vi "FEA_Model_LEMP.vi"(8 "error in (no error)":errorcluster, 11 "FEA_Model in":refnum<class "FEA_Model.lvclass">) -> (0 "error out":errorcluster, 3 "FEA_Model out":refnum<class "FEA_Model.lvclass">)   [LabVIEW 2021, in "FEA_Model.lvclass"]
uses:
  FEA_Model.lvclass
  FEA_Model.lvclass/FEA_Model.ctl
panel:
  in  "Mode count":i32=3
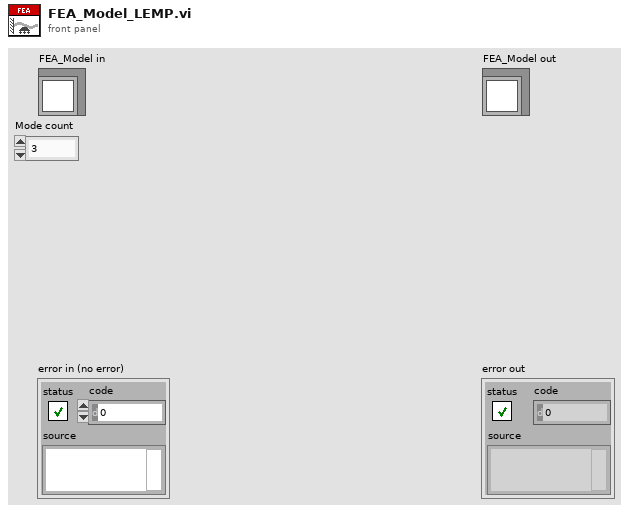
[diagram p1: front panel]
types:
  T1 = cluster{"Eigenvalues":dbl[], "SquareT Eigenvectors":dbl[][], "1/deltaStiff":dbl}
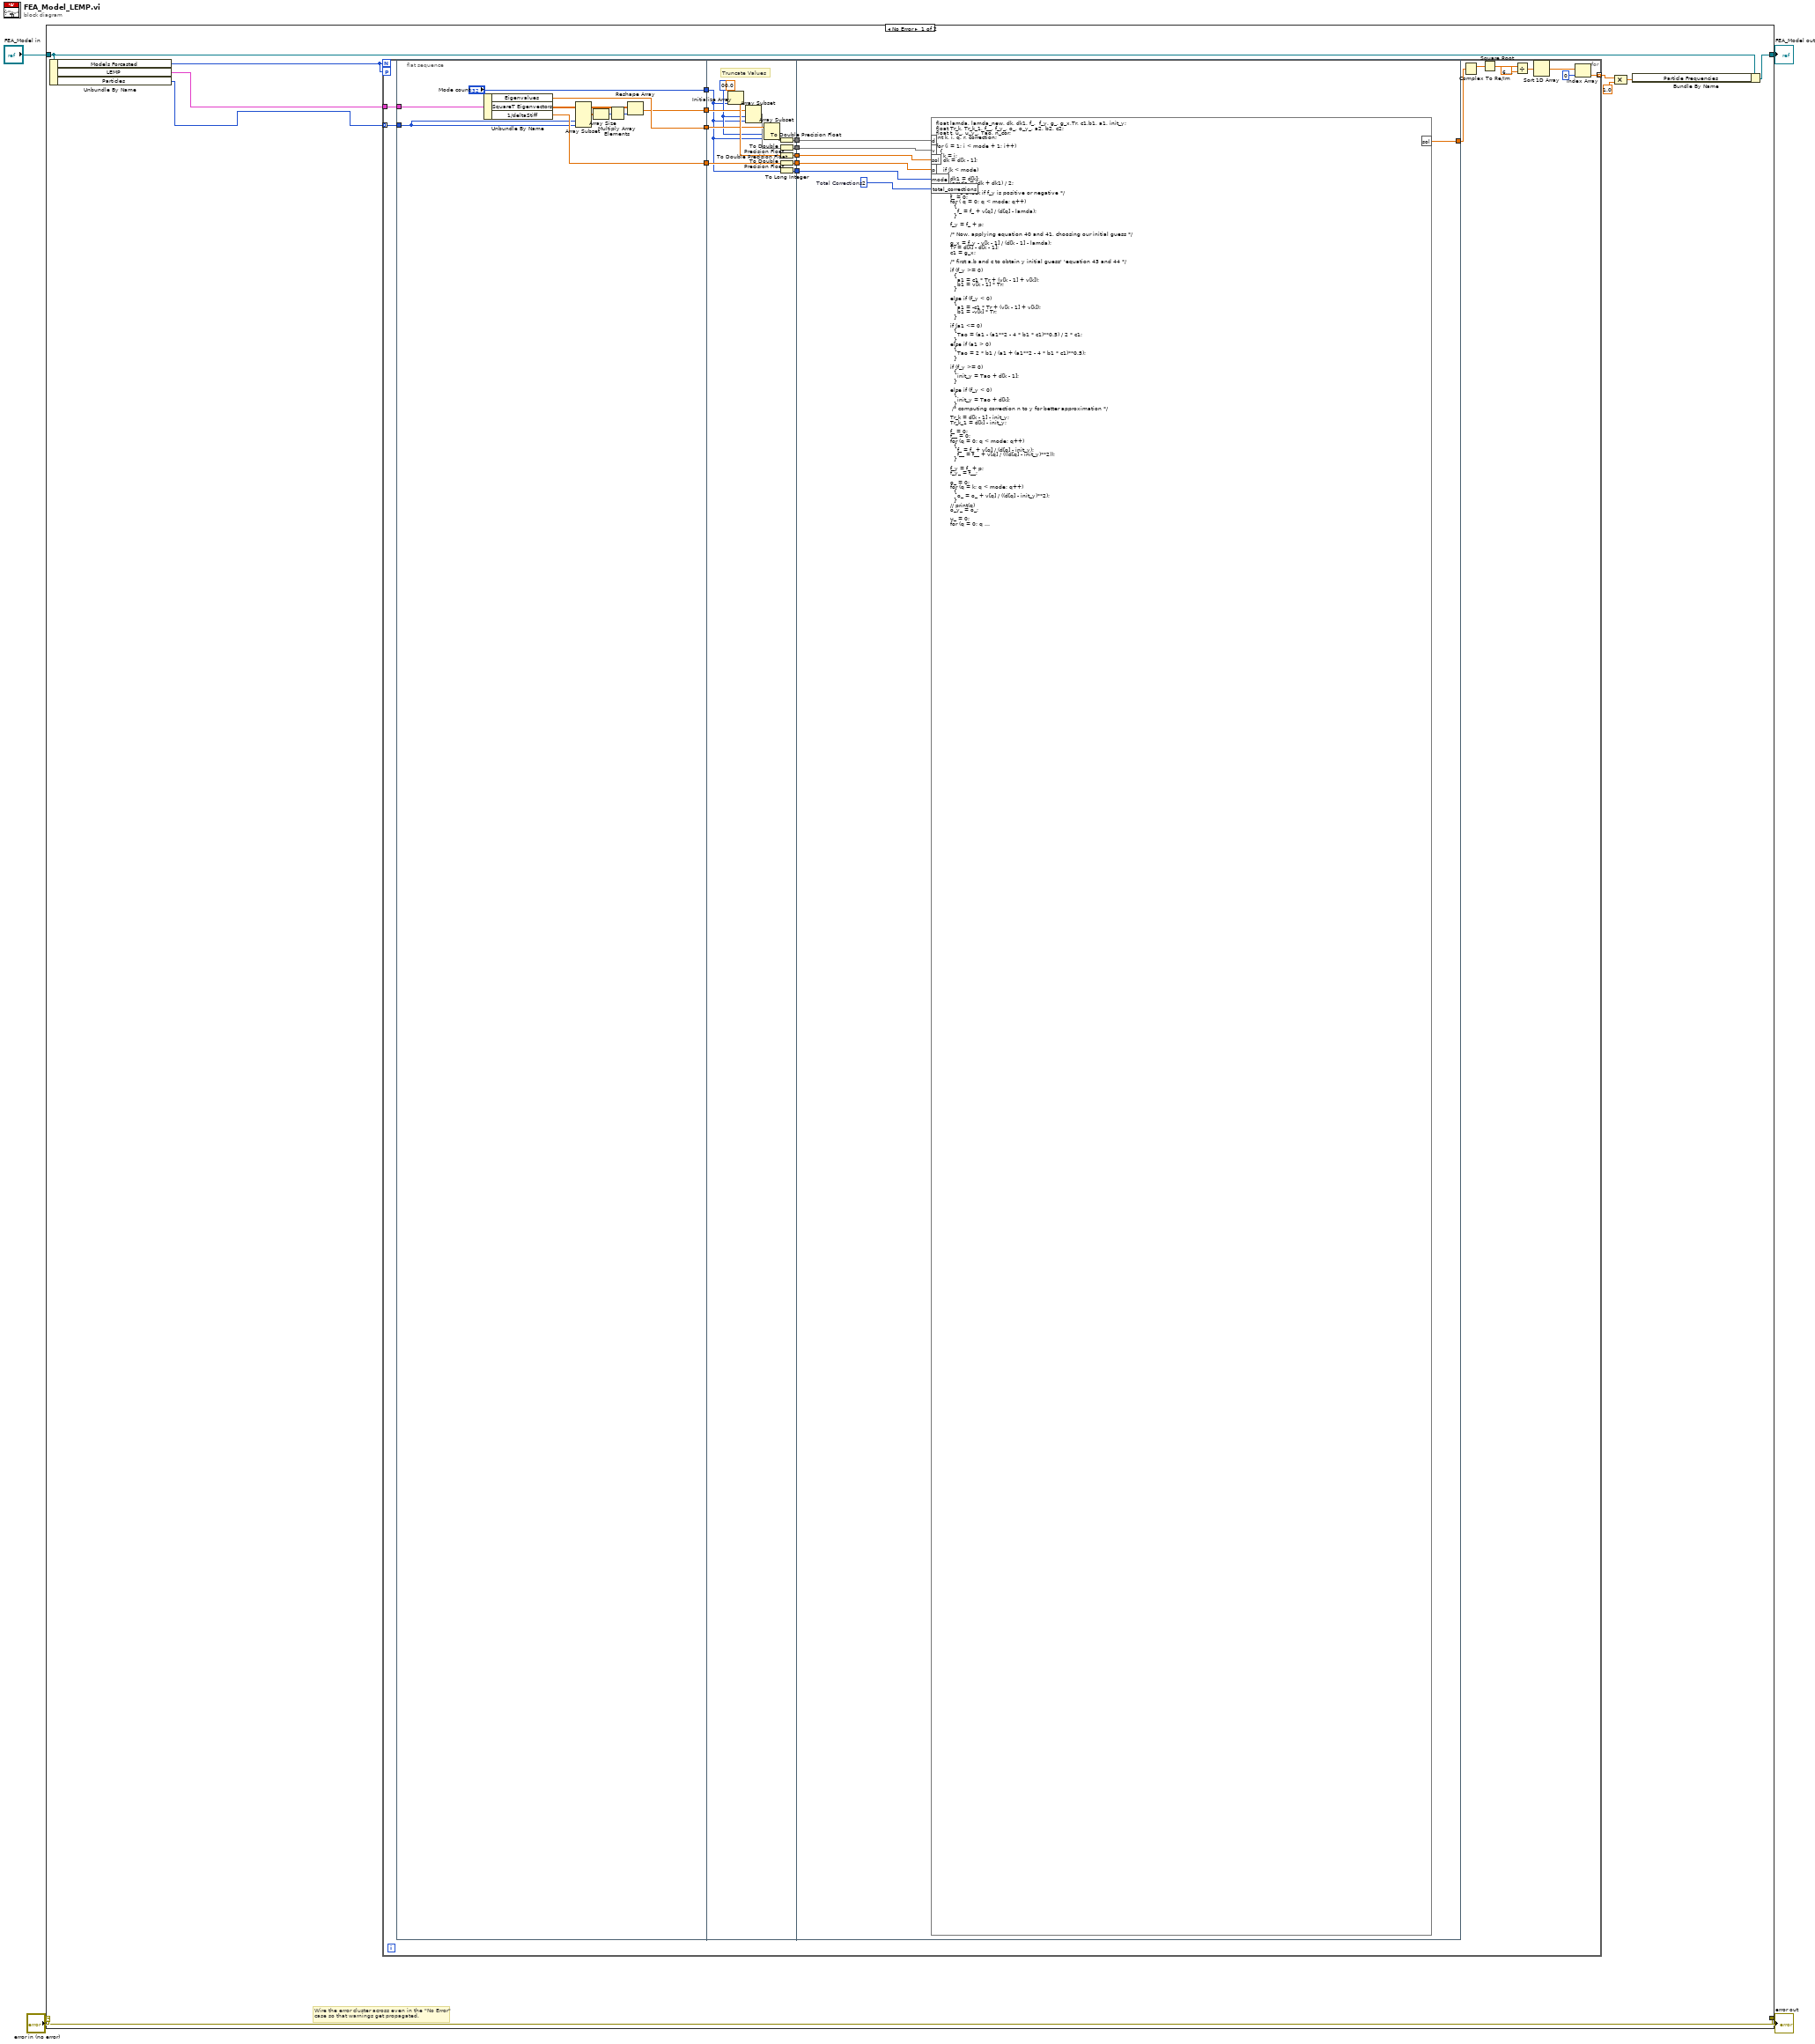
[diagram p0: block diagram]
diagram:
  n1 = case shown="No Error" "error in (no error)" {
    selector: "error in (no error)" -> [w13 w65]
    tunnel: [w13 w65] -> w3
    tunnel: "FEA_Model in" -> [w11 w64]
    tunnel: [w10 w64] -> w1
    frame No Error {
      # "Wire the error cluster across even in the \"No Error\"\ncase so that warnings get propagated."
      n2 = Unbundle By Name(w11) -> ("Models Forcasted"=w9:i32, "LEMP"=w12:T1, "Particles"=w5:i32[])
      n3 = for {
        N: w9 -> [_]
        tunnel: w5 -> [w23] mode=indexing
        tunnel: w12 -> [w22]
        workers-P: w9 -> [_]
        tunnel: [w14] -> w8 mode=indexing
        n4 = flat-sequence {
          tunnel: [w36] -> w32
          tunnel: [w38] -> w31
          tunnel: [w37] -> w30
          tunnel: ["Mode count"] -> w29
          tunnel: w23 -> [w34]
          tunnel: w22 -> [w35]
          tunnel: [w48] -> w28
          tunnel: [w46] -> w27
          tunnel: [w44] -> w25
          tunnel: [w45] -> w24
          tunnel: [w43] -> w26
          tunnel: w32 -> [w53]
          tunnel: w31 -> [w52]
          tunnel: w30 -> [w56]
          tunnel: w29 -> [w47]
          tunnel: w28 -> [w63]
          tunnel: w27 -> [w62]
          tunnel: w26 -> [w59]
          tunnel: w25 -> [w60]
          tunnel: w24 -> [w61]
          tunnel: [w58] -> w15
          frame #0 {
            n5 = Unbundle By Name(w35) -> ("Eigenvalues"=w38:dbl[], "SquareT Eigenvectors"=w42:dbl[][], "1/deltaStiff"=w37:dbl)
            n6 = Array Subset(array=w42, index (col)=w34, length (col)=w34) -> (w41:dbl[][])  [unwired: 2 in]
            n7 = Array Size(array=w41) -> (size(s)=w39:i32[])
            n8 = Multiply Array Elements(1:w39) -> (0:w40:i32)
            n9 = Reshape Array(w41, w40) -> (w36:dbl[])
          }
          frame #1 {
            w50 = 0
            # "Truncate Values"
            n10 = Initialize Array(0.0, w47) -> (w54:dbl[])
            n11 = Array Subset(array=w53, index=w50, length=w47) -> (w51:dbl[])
            n12 = Array Subset(array=w52, index=w50, length=w47) -> (w49:dbl[])
            n13 = To Double Precision Float(number=w49) -> (double precision float=w48:dbl[])
            n14 = To Double Precision Float(number=w51) -> (double precision float=w46:dbl[])
            n15 = To Double Precision Float(number=w54) -> (double precision float=w45:dbl[])
            n16 = To Double Precision Float(number=w56) -> (double precision float=w44:dbl)
            n17 = To Long Integer(number=w47) -> (32bit integer=w43:i32)
          }
          frame #2 {
            w57 = 2  # Total Corrections
            n18 = formula code="float lamda, lamda_new, dk, dk1, f_,  f_y, g_, g_x,Tr, c1,b1, a1, init_y;\nfloat Tr_k, Tr_k_1, f__, f_y_, o_, o_y_, a2, b2, c2;\nfloat t, u_, u_y_, Tao, n_cor;\nint k, i, q, r, correction;\n\nfor (i = 1; i < mode + 1; i++)\n  {\n    k = i;\n    dk = d[k - 1];\n\n    if (k < mode)\n      {\n        dk1 = d[k];\n        lamda = (dk + dk1) / 2;\n\n        /* To check if f_y is positive or negative */\n        f_ = 0;\n        for ( q = 0; q < mode; q++)\n          {\n            f_ = f_ + v[q] / (d[q] - lamda);\n          }\n\n        f_y = f_ + p;\n\n        /* Now, applying equation 40 and 41, choosing our initial guess */\n\n        g_x = f_y - v[k - 1] / (d[k - 1] - lamda);\n        Tr = d[k] - d[k - 1];\n        c1 = g_x;\n\n        /* first a,b and c to obtain y initial guess' 'equation 43 and 44 */\n\n        if (f_y >= 0)\n          {\n            a1 = c1 * Tr + (v[k - 1] + v[k]);\n            b1 = v[k - 1] * Tr;\n          }\n\n        else if (f_y < 0)\n          {\n            a1 = -c1 * Tr + (v[k - 1] + v[k]);\n            b1 = -v[k] * Tr;\n          }\n\n        if (a1 <= 0)\n          {\n            Tao = (a1 - (a1**2 - 4 * b1 * c1)**0.5) / 2 * c1;\n          }\n        else if (a1 > 0)\n          {\n            Tao = 2 * b1 / (a1 + (a1**2 - 4 * b1 * c1)**0.5);\n          }\n\n        if (f_y >= 0)\n          {\n            init_y = Tao + d[k - 1];\n          }\n\n        else if (f_y < 0)\n          {\n            init_y = Tao + d[k];\n          }\n         /* computing correction n to y for better approximation */\n\n        Tr_k = d[k - 1] - init_y;\n        Tr_k_1 = d[k] - init_y;\n\n        f_ = 0;\n        f__ = 0;\n        for (q = 0; q < mode; q++)\n          {\n            f_ = f_ + v[q] / (d[q] - init_y);\n            f__ = f__ + v[q] / (((d[q] - init_y)**2));\n          }\n\n        f_y = f_ + p;\n        f_y_ = f__;\n\n        o_ = 0;\n        for (q = k; q < mode; q++)\n          {\n            o_ = o_ + v[q] / ((d[q] - init_y)**2);\n          }\n        // print(q)\n        o_y_ = o_;\n\n        u_ = 0;\n        for (q = 0; q < mode; q++)\n          {\n            u_ = u_ + v[q] / ((d[q] - init_y)**2);\n          }\n        // print(q)\n\n        u_y_ = u_;\n        /*'second a, b and c for final correction' */\n\n        a2 = (Tr_k + Tr_k_1) * f_y - Tr_k * Tr_k_1 * f_y_;\n        b2 = Tr_k * Tr_k_1 * f_y;\n\n        if (f_y >= 0)\n          {\n            c2 = f_y - Tr_k_1 * f_y_ - u_y_ * (d[k - 1] - d[k]);\n          }\n\n        else if (f_y < 0)\n          {\n            c2 = f_y - Tr_k * f_y_ - o_y_ * (d[k] - d[k - 1]);\n          }\n\n        if (a2 <= 0)\n          {\n            n_cor = (a2 - (a2**2 - 4 * b2 * c2)**0.5) / 2 * c2;\n          }\n\n        else if (a2 > 0)\n          {\n            n_cor = 2 * b2 / (a2 + (a2**2 - 4 * b2 * c2)**0.5);\n          }\n\n        lamda_new = init_y + n_cor;\n        /*computing second correction n to y for better approximation */\n        // init_y = lamda_new;\n\n        sol[k - 1] = lamda_new;\n      }\n\n    else if (k == mode)\n      {\n        t = 0;\n        for (r = 0; r < mode; r++)\n          {\n            t = t + (v[r]**2);\n          }\n\n        float d6;\n\n        d6 = d[k - 1] + t / p;\n\n        lamda = (d6 + d[k - 1]) / 2;\n\n        //'To check if f_y is positive or negative'\n\n        f_ = 0;\n        for( q = 0; q < mode; q++)\n          {\n            f_ = f_ + v[q] / (d[q] - lamda);\n          }\n\n        f_y = f_ + p;\n\n        //'Now, applying equation 40 and 41, choosing our initial guess'\n        /*g_ = 0;\n           for( q = 0; q<n; q++)\n           {\n           g_ = g_ + v[q]/(d[q]-lamda);\n           }\n\n           g_x = g_ + p; */\n\n        g_x = f_y - v[k - 1] / (d[k - 1] - lamda);\n        Tr = d[k - 1] - d[k - 2];\n        c1 = g_x;\n\n        //'first a,b and c to obtain y initial guess' 'equation 43 and 44'\n        if (f_y <= 0)\n          {\n            a1 = c1 * Tr + (v[k - 2] + v[k - 1]);\n            b1 = v[k - 1] * Tr;\n          }\n\n        else if (f_y > 0)\n          {\n            a1 = -c1 * Tr + (v[k - 2] + v[k - 1]);\n            b1 = -v[k - 1] * Tr;\n          }\n\n        if (a1 <= 0)\n          {\n            Tao = (a1 + (a1**2 - 4 * b1 * c1)**0.5) / 2 * c1;\n          }\n\n        else if (a1 > 0)\n          {\n            Tao = 2 * b1 / (a1 - (a1**2 - 4 * b1 * c1)**0.5);\n          }\n\n        init_y = Tao + d[k - 1];\n\n        //'computing correction n to y for better approximation'\n        for (correction = 1; correction < total_corrections; correction++)\n          {\n\n            Tr_k = d[k - 1] - init_y;\n            Tr_k_1 = d6 - init_y;\n\n            f_ = 0;\n            f__ = 0;\n            for (q = 0; q < mode; q++)\n              {\n                f_ = f_ + v[q] / (d[q] - init_y);\n                f__ = f__ + v[q] / ((d[q] - init_y)**2);\n              }\n\n            f_y = f_ + p;\n            f_y_ = f__;\n\n            u_ = 0;\n            for (q = 0; q < mode; q++)\n              {\n                u_ = u_ + v[q] / ((d[q] - init_y)**2);\n              }\n\n            u_y_ = u_;\n            //'second a, b and c for final correction'\n\n            a2 = (Tr_k + Tr_k_1) * f_y - Tr_k * Tr_k_1 * f_y_;\n            b2 = Tr_k * Tr_k_1 * f_y;\n            c2 = f_y - Tr_k * u_y_ - (v[k - 1] / Tr_k_1);\n\n            if (a2 <= 0)\n              {\n                n_cor = (a2 - (a2**2 - 4 * b2 * c2)**0.5) / 2 * c2;\n              }\n\n            else if (a2 > 0)\n              {\n                n_cor = 2 * b2 / (a2 + (a2**2 - 4 * b2 * c2)**0.5);\n              }\n\n            lamda_new = init_y + n_cor;\n            init_y = lamda_new;\n          }\n        sol[mode - 1] = lamda_new;\n      }\n  }"("d"=w63, "v"=w62, "p"=w60, "mode"=w59, "sol"=w61, "total_corrections"=w57) -> ("sol"=w58:dbl[])
          }
        }
        n19 = Complex To Re/Im ("Complex To Cartesian.vi")(x + iy=w15) -> (x=w21:dbl[])  [unwired: 1 out]
        n20 = Square Root ("Square Root.vi")(x=w21) -> (sqrt(x)=w20:dbl[])
        n21 = Divide(x=w20, y=6.283185307179586) -> (x/y=w16:dbl[])
        n22 = Sort 1D Array(array=w16) -> (sorted array=w18:dbl[])
        n23 = Index Array(array=w18, index=0) -> (element=w14:dbl)
      }
      n24 = Compound Arithmetic op=MULTIPLY(w8, 1.0) -> (w7:dbl[])
      n25 = Bundle By Name(cluster=w11, "Particle Frequencies"=w7) -> (w10:refnum<class "FEA_Model.lvclass">)
    }
    frame Error {
    }
  }
  "error out" <- w3
  "FEA_Model out" <- w1
